vi "Train ramp (No Objects).vi"(7 "Cluster In":T4={"Field"=0.0, "Rate"=0.0, "Status"={"Sweeping"=FALSE, "Clamped"=FALSE, "Hold"=FALSE, "At Rest"=FALSE, "Quench"=FALSE, "Persistent Mode"=FALSE, "Switch Heater"=FALSE}, "ILM Shut Down?"=FALSE, "IO Info"={"Address"={"Com Port"=1, "ISOBUS Address"=2, "GPIB Address"=24, "Communication"=enum."ISOBUS"}, "Version"=enum."IPS"}, "IO Info (Level Meter)"={"Address"={"Com Port"=1, "ISOBUS Address"=5, "GPIB Address"=24, "Communication"=enum."ISOBUS"}, "ILM Name"="", "Display Channel"=[]}, "Training?"=FALSE, "Training Field and Speed Cluster"={"Training Field"=[0.0, 4.108, 5.78, 8.001], "Training Speed"=[0.0057, 0.0022833333333333334, 0.0011333333333333334, 0.0011333333333333334]}}, 9 "input":dbl[unit], 11 "field":dbl[unit]) -> (0 "output":dbl[unit], 2 "change?":bool, 3 "Cluster Out":T4={"Field"=0.0, "Rate"=0.0, "Status"={"Sweeping"=FALSE, "Clamped"=FALSE, "Hold"=FALSE, "At Rest"=FALSE, "Quench"=FALSE, "Persistent Mode"=FALSE, "Switch Heater"=FALSE}, "ILM Shut Down?"=FALSE, "IO Info"={"Address"={"Com Port"=1, "ISOBUS Address"=2, "GPIB Address"=24, "Communication"=enum."ISOBUS"}, "Version"=enum."IPS"}, "IO Info (Level Meter)"={"Address"={"Com Port"=1, "ISOBUS Address"=5, "GPIB Address"=24, "Communication"=enum."ISOBUS"}, "ILM Name"="", "Display Channel"=[]}, "Training?"=FALSE, "Training Field and Speed Cluster"={"Training Field"=[0.0, 4.108, 5.78, 8.001], "Training Speed"=[0.0057, 0.0022833333333333334, 0.0011333333333333334, 0.0011333333333333334]}})   [LabVIEW 2012]
uses:
  Magnet status.ctl
  Oxford/PSSUBS.LLB/PSIO.ctl
  Oxford/BUSGEN.LLB/OxfordAddress.ctl
  Power Supply.lvclass
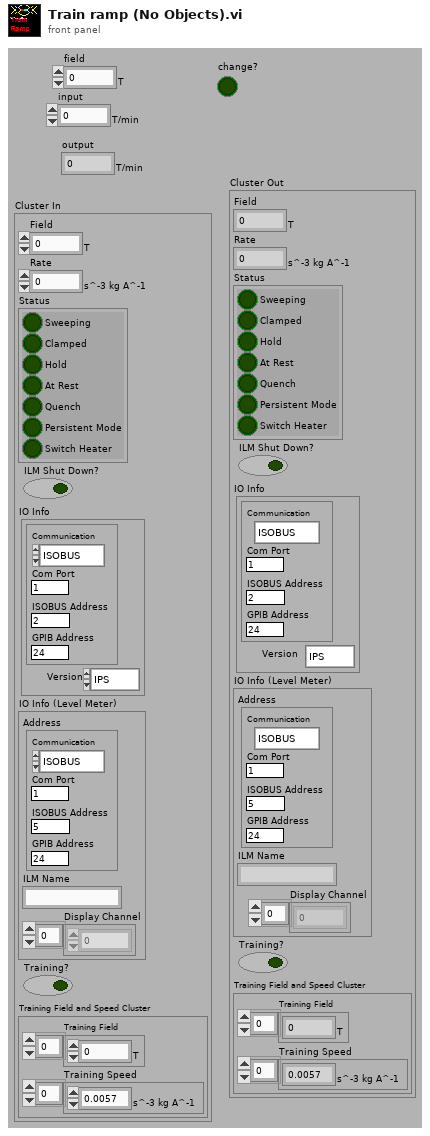
[diagram p1: front panel]
types:
  T1 = typedef "Power Supply.lvclass/Magnet status.ctl" = cluster{"Sweeping":bool, "Clamped":bool, "Hold":bool, "At Rest":bool, "Quench":bool, "Persistent Mode":bool, "Switch Heater":bool}
  T2 = typedef "PSIO.ctl" = cluster{"Address":T3, "Version":enum16{"PS", "IPS"}}
  T3 = typedef "OxfordAddress.ctl" = cluster{"Com Port":i32, "ISOBUS Address":i32, "GPIB Address":i16, "Communication":enum16{"RS232", "ISOBUS", "GPIB", "Gateway"}}
  T4 = cluster{"Field":dbl[unit], "Rate":dbl[unit], "Status":T1, "ILM Shut Down?":bool, "IO Info":T2, "IO Info (Level Meter)":cluster{"Address":T3, "ILM Name":string, "Display Channel":i32[]}, "Training?":bool, "Training Field and Speed Cluster":cluster{"Training Field":dbl[unit][], "Training Speed":dbl[unit][]}}
  T5 = cluster{"Training Field":dbl[unit][], "Training Speed":dbl[unit][]}
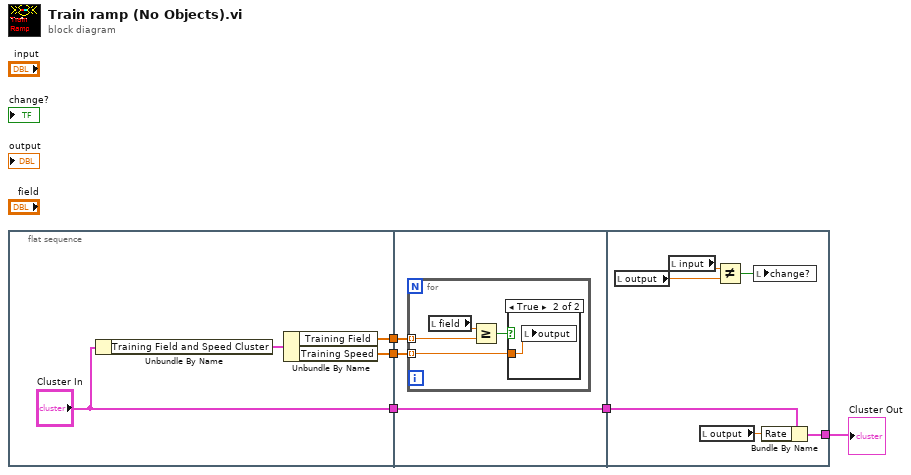
[diagram p0: block diagram]
diagram:
  n1 = flat-sequence {
    tunnel: [w8] -> w5
    tunnel: [w7] -> w4
    tunnel: ["Cluster In"] -> w3
    tunnel: w5 -> [w12]
    tunnel: w4 -> [w11]
    tunnel: w3 -> [w10]
    tunnel: [w10] -> w2
    tunnel: w2 -> [w23]
    tunnel: [w21] -> w1
    frame #0 {
      n2 = Unbundle By Name("Cluster In") -> ("Training Field and Speed Cluster"=w9:T5)
      n3 = Unbundle By Name(w9) -> ("Training Field"=w8:dbl[unit][], "Training Speed"=w7:dbl[unit][])
    }
    frame #1 {
      n4 = for {
        tunnel: w12 -> [w15] mode=indexing
        tunnel: w11 -> [w13] mode=indexing
        n5 = local read "field"() -> (w16:dbl[unit])
        n6 = Greater Or Equal?(x=w16, y=w15) -> (x >= y?=w14:bool)
        n7 = case shown="True" w14 {
          tunnel: w13 -> [_ w17]
          frame False {
          }
          frame True {
            n8 = local write "output"(w17) -> ()
          }
        }
      }
    }
    frame #2 {
      n9 = local read "output"() -> (w19:dbl[unit])
      n10 = local read "input"() -> (w20:dbl[unit])
      n11 = local read "output"() -> (w22:dbl[unit])
      n12 = Not Equal?(x=w20, y=w19) -> (x != y?=w18:bool)
      n13 = local write "change?"(w18) -> ()
      n14 = Bundle By Name(cluster=w23, "Rate"=w22) -> (w21:T4)
    }
  }
  "Cluster Out" <- w1
